vi "PIEZO_standard_init.vi"(2 "Incoming Handle":i32, 3 "error in":errorcluster) -> (0 "Outgoing Handle":i32, 1 "error out":errorcluster)   [LabVIEW 2015]
uses:
  <userlib>/Madlib.dll
panel:
  # "This VI implements an initialization sequence for use with \na single Nano-Drive."
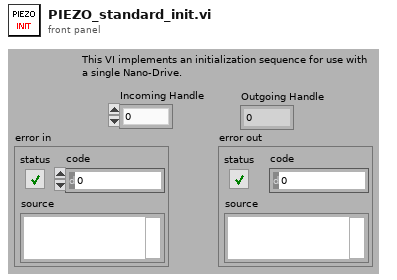
[diagram p1: front panel]
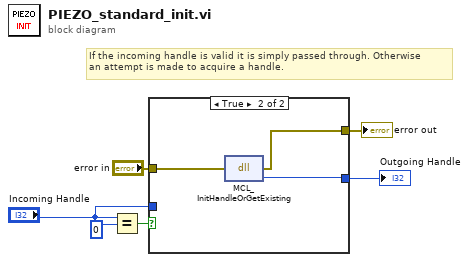
[diagram p0: block diagram]
diagram:
  # "If the incoming handle is valid it is simply passed through. Otherwise\nan attempt is made to acquire a handle."
  n1 = Equal?(x="Incoming Handle", y=0) -> (x = y?=w5:bool)
  n2 = case shown="True" w5 {
    tunnel: [w8 w11] -> w3
    tunnel: "Incoming Handle" -> [w8 _]
    tunnel: "error in" -> [w7 w10]
    tunnel: [w7 w9] -> w1
    frame False {
    }
    frame True {
      n3 = dll-call lib="C:/Program Files/National Instruments/LabVIEW 2015/user.lib/Madlib.dll" fn="MCL_InitHandleOrGetExisting"(error in=w10) -> (error out=w9:errorcluster, "return type"=w11:i32)  [unwired: 2 in, 1 out]
    }
  }
  "Outgoing Handle" <- w3
  "error out" <- w1
